vi "FTW-Connector-Ask.vi"(0 "FTW Actor Connector":refnum<class "FTW-ActorConnector.lvclass">, 5 "Request Header":string, 7 "Request Body":string, 9 "Timeout":i32=100 format="%dmsec", 11 "error in":errorcluster) -> (4 "FTW Actor Connector out":refnum<class "FTW-ActorConnector.lvclass">, 6 "Response Header":string, 8 "Response Body":string, 10 "Timed out?":bool, 15 "error out":errorcluster)   [LabVIEW 2013, in "FTW-Actor.lvlib" / "FTW-ActorConnector.lvclass"]
uses:
  FTW-ActorConnector.lvclass
  FTW-ActorConnector.lvclass/FTW-ActorConnector.ctl
  Endpoint/FTW-Endpoint.lvclass
panel:
  # "Inputs"
  # "Outputs"
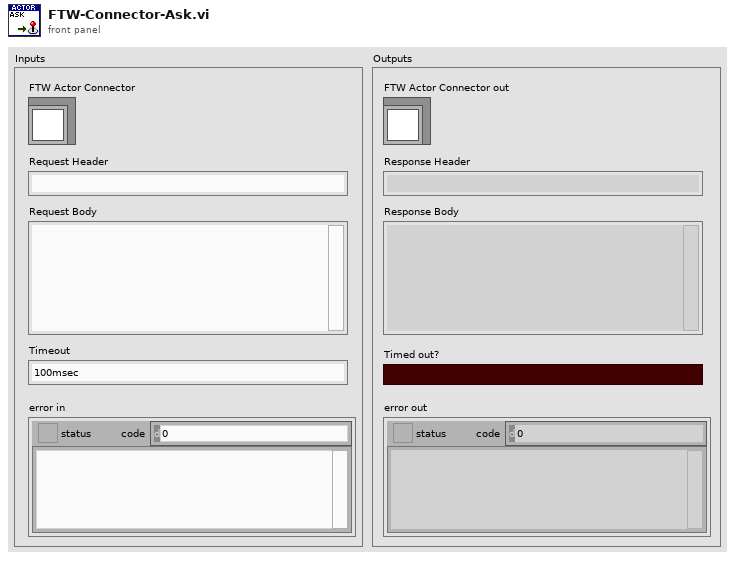
[diagram p1: front panel]
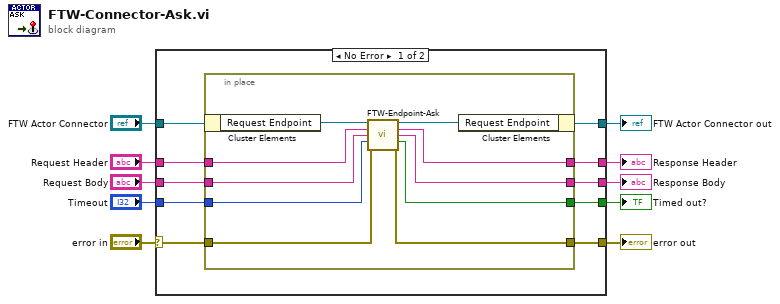
[diagram p0: block diagram]
diagram:
  n1 = case shown="No Error" "error in" {
    selector: "error in" -> [w19 w32]
    tunnel: [w17 w32] -> w9
    tunnel: "FTW Actor Connector" -> [w20 w31]
    tunnel: [w18 w31] -> w7
    tunnel: "Request Header" -> [w16 _]
    tunnel: "Request Body" -> [w15 _]
    tunnel: [w14 _] -> w6
    tunnel: "Timeout" -> [w13 _]
    tunnel: [w12 _] -> w2
    tunnel: [w11 _] -> w1
    frame No Error {
      n2 = in-place {
        in-place-border: w19 -> [w30]
        in-place-border: [w29] -> w17
        in-place-border: w16 -> [w25]
        in-place-border: w15 -> [w24]
        in-place-border: [w26] -> w14
        in-place-border: w13 -> [w23]
        in-place-border: [w22] -> w12
        in-place-border: [w21] -> w11
        n3 = in-place-cluster #1(w20) -> ("Request Endpoint"=w28:refnum<class "FTW-Endpoint.lvclass">)
        n4 = call-dynamic "FTW-Endpoint-Ask.vi"("FTW Socket"=w28, "Request Header"=w25, "Request Body"=w24, "Timeout"=w23, "error in"=w30) -> ("FTW Socket out"=w27:refnum<class "FTW-Endpoint.lvclass">, "Response Header"=w22:string, "Response Body"=w21:string, "Timed out?"=w26:bool, "error out"=w29:errorcluster)  [unwired: 6 in]
        n5 = in-place-cluster #1("Request Endpoint"=w27) -> (w18:refnum<class "FTW-ActorConnector.lvclass">)
      }
    }
    frame Error {
    }
  }
  "error out" <- w9
  "FTW Actor Connector out" <- w7
  "Timed out?" <- w6
  "Response Header" <- w2
  "Response Body" <- w1
